vi "dvr_fgv_map_write.vi"(8 "error in (no error)":errorcluster, 11 "value":variant) -> (0 "error out":errorcluster)   [LabVIEW 2020]
uses:
  map_state.ctl
  <vilib>/Utility/miscctls.llb/LVMapReplaceAction.ctl
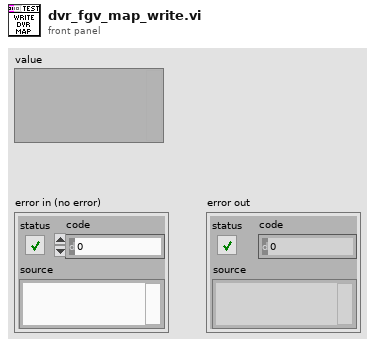
[diagram p1: front panel]
types:
  T1 = typedef "map_state.ctl" = enum16{"flag"}
  T2 = typedef "LVMapReplaceAction.ctl" = enum32{"Modify Entry only if found", "Add or Modify Entry", "Delete Entry"}
  T3 = typedef "ram_state.ctl" = enum16{"flag"}
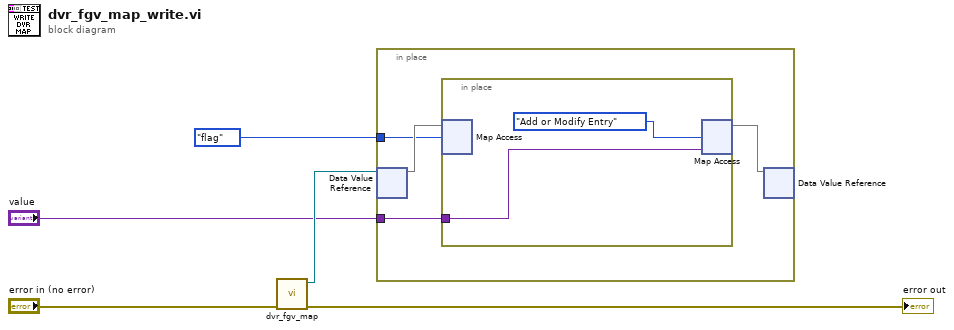
[diagram p0: block diagram]
diagram:
  n1 = call "dvr_fgv_map.vi"("error in (no error)"="error in (no error)") -> ("error out"=→"error out":errorcluster, "data value reference"=w3:refnum<data-value>)  [unwired: 9 in]
  n2 = in-place {
    in-place-border: map_state."flag" ("key") -> [w8]
    in-place-border: "value" -> [w6]
    n3 = in-place-dvr #1(w3) -> (w9:map{T3, variant})  [unwired: 1 out]
    n4 = in-place {
      in-place-border: w6 -> [w10]
      n5 = in-place-map #2(w9, w8) -> ()  [unwired: 1 in, 2 out]
      n6 = in-place-map #2(w10, LVMapReplaceAction."Add or Modify Entry" ("action")) -> (w7:map{T3, variant})  [unwired: 2 out]
    }
    n7 = in-place-dvr #1(w7) -> ()  [unwired: 2 out]
  }
